vi "VDH-calcCalibrationFactors.vi"(8 "error in (no error)":errorcluster, 11 "VDH-VNA_data_handler in":refnum<class "VDH-VNA_data_handler.lvclass">) -> (0 "error out":errorcluster, 3 "VDH-VNA_data_handler out":refnum<class "VDH-VNA_data_handler.lvclass">)   [LabVIEW 2020, in "VDH-VNA_data_handler.lvlib" / "VDH-VNA_data_handler.lvclass"]
uses:
  VDH-VNA_data_handler.lvclass
  VDH-Calibration_enum.ctl
  VDH-VNA_data_handler.lvclass/VDH-VNA_data_handler.ctl
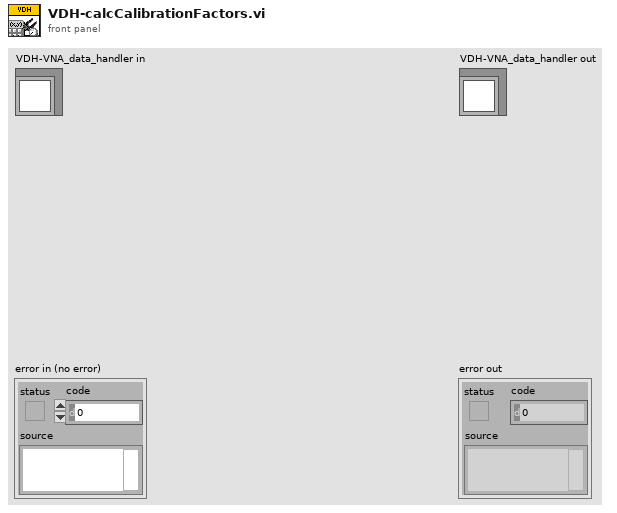
[diagram p1: front panel]
types:
  T1 = typedef "VDH-VNA_data_handler.lvlib/VDH-VNA_data_handler.lvclass/VDH-Calibration_enum.ctl" = enum16{"Non", "Short", "Open", "Load", "Through", "Permativity"}
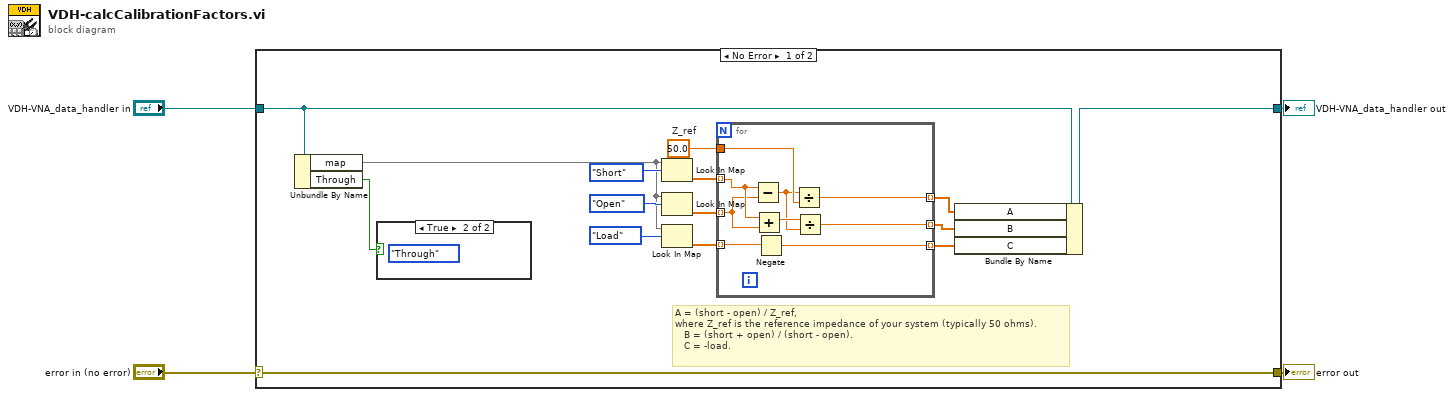
[diagram p0: block diagram]
diagram:
  n1 = case shown="No Error" "error in (no error)" {
    selector: "error in (no error)" -> [w19 w30]
    tunnel: [w19 w30] -> w3
    tunnel: [w8 w29] -> w1
    tunnel: "VDH-VNA_data_handler in" -> [w18 w29]
    frame No Error {
      w9 = 50.0  # Z_ref
      # "A = (short - open) / Z_ref, \nwhere Z_ref is the reference impedance of your system (typically 50 ohms).\n\t\t B = (short + open) / (short - open).\n   C = -load."
      n2 = Unbundle By Name(w18) -> ("map"=w14:map{T1, cdb[]}, "Through"=w17:bool)
      n3 = case shown="True" w17 {
        frame False {
        }
        frame True {
          (unwired) VDH-Calibration_enum."Through" ("SOLT")
        }
      }
      n4 = Look In Map(map=w14, key=VDH-Calibration_enum."Short" ("SOLT")) -> (value=w12:cdb[])  [unwired: 1 in, 1 out]
      n5 = Look In Map(map=w14, key=VDH-Calibration_enum."Open" ("SOLT")) -> (value=w11:cdb[])  [unwired: 1 in, 1 out]
      n6 = Look In Map(map=w14, key=VDH-Calibration_enum."Load" ("SOLT")) -> (value=w10:cdb[])  [unwired: 1 in, 1 out]
      n7 = for {
        tunnel: w12 -> [w26] mode=indexing
        tunnel: w11 -> [w25] mode=indexing
        tunnel: w10 -> [w27] mode=indexing
        tunnel: w9 -> [w28]
        tunnel: [w24] -> w5 mode=indexing
        tunnel: [w21] -> w6 mode=indexing
        tunnel: [w20] -> w7 mode=indexing
        n8 = Subtract(x=w26, y=w25) -> (x-y=w22:cdb)
        n9 = Add(x=w26, y=w25) -> (x+y=w23:cdb)
        n10 = Negate(x=w27) -> (-x=w20:cdb)
        n11 = Divide(x=w22, y=w28) -> (x/y=w24:cdb)
        n12 = Divide(x=w23, y=w22) -> (x/y=w21:cdb)
      }
      n13 = Bundle By Name(cluster=w18, "A"=w5, "B"=w6, "C"=w7) -> (w8:refnum<class "VDH-VNA_data_handler.lvclass">)
    }
    frame Error {
    }
  }
  "error out" <- w3
  "VDH-VNA_data_handler out" <- w1
